vi "Format Power No Objects.vi"(8 "error in":errorcluster, 9 "Precision":u16=3, 10 "Power":dbl, 11 "Cluster In":T2={"Wavelength"=0.0, "AVG"=0, "Range"=0, "Backlight"=0, "Beeper"=0, "Zero"=0, "Local Lockout"=0, "ATTN"=0, "Run/Stop"=0, "Units"=0, "Averaging Time"=0.5, "Averaging"=FALSE, "Most Recent Power"=5.5, "Filter"=1} {"AVG" items=["Slow"=1, "Medium"=2, "Fast"=3]; "Range" items=["Auto", "Lowest", "2", "3", "4", "5", "6", "7", "Highest"]; "Backlight" items=["Off", "Low", "High"]; "Beeper" items=["Off", "On"]; "Zero" items=["Off", "On"]; "Local Lockout" items=["Off", "On"]; "ATTN" items=["Off", "On"]; "Run/Stop" items=["Stop", "Run"]; "Units" items=["W"=1, "dB"=2, "dBm"=3, "REL"=4]; "Filter" items=["Orange"=1, "Green"=2, "Yellow"=3]}) -> (0 "error out":errorcluster, 2 "Formatted Power":string, 3 "Cluster Out":T2={"Wavelength"=0.0, "AVG"=0, "Range"=0, "Backlight"=0, "Beeper"=0, "Zero"=0, "Local Lockout"=0, "ATTN"=0, "Run/Stop"=0, "Units"=0, "Averaging Time"=0.5, "Averaging"=FALSE, "Most Recent Power"=5.5, "Filter"=1} {"AVG" items=["Slow"=1, "Medium"=2, "Fast"=3]; "Range" items=["Auto", "Lowest", "2", "3", "4", "5", "6", "7", "Highest"]; "Backlight" items=["Off", "Low", "High"]; "Beeper" items=["Off", "On"]; "Zero" items=["Off", "On"]; "Local Lockout" items=["Off", "On"]; "ATTN" items=["Off", "On"]; "Run/Stop" items=["Stop", "Run"]; "Units" items=["W"=1, "dB"=2, "dBm"=3, "REL"=4]; "Filter" items=["Orange"=1, "Green"=2, "Yellow"=3]})   [LabVIEW 2012]
doc: "Formats the provided power with current units of Power Meter Object.\nEx.\n.000253 --> 253uW"
uses:
  Newport 1830-C/Public/Filters.ctl
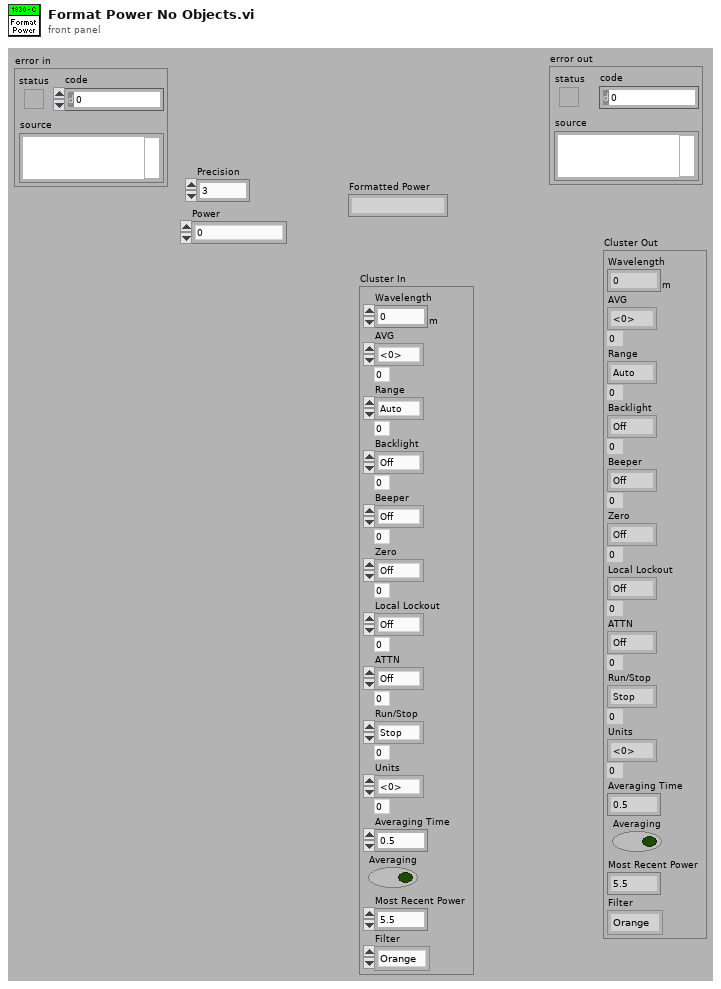
[diagram p1: front panel]
types:
  T1 = typedef "Filters.ctl" = u16
  T2 = cluster{"Wavelength":dbl[unit], "AVG":u16, "Range":u16, "Backlight":u16, "Beeper":u16, "Zero":u16, "Local Lockout":u16, "ATTN":u16, "Run/Stop":u16, "Units":u16, "Averaging Time":dbl, "Averaging":bool, "Most Recent Power":dbl, "Filter":T1}
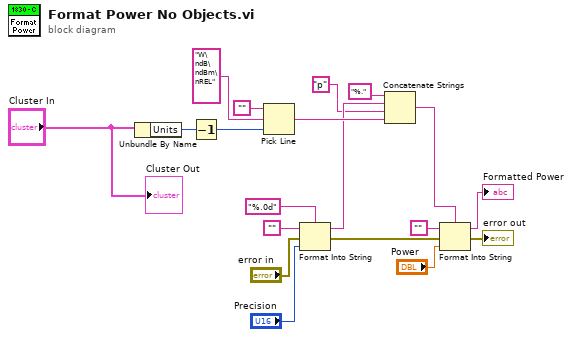
[diagram p0: block diagram]
diagram:
  n1 = Unbundle By Name("Cluster In") -> ("Units"=w14:u16)
  n2 = Decrement(x=w14) -> (x-1=w13:u16)
  n3 = Pick Line(string ("")="", multi-line string="W\ndB\ndBm\nREL", line index=w13) -> (output string=w11:string)
  n4 = Format Into String(format string="%.0d", initial string="", error in="error in", "Precision") -> (resulting string=w4:string, error out=w6:errorcluster)
  n5 = Concatenate Strings("%." ("string"), w4, "p" ("string"), w11) -> (w19:string)
  n6 = Format Into String(format string=w19, initial string="", error in=w6, "Power") -> (resulting string=→"Formatted Power":string, error out=→"error out":errorcluster)
  "Cluster Out" <- "Cluster In"
